vi "Quick Start - Runs - Get.vi"() -> ()   [LabVIEW 2020]
uses:
  Nominal Client/Nominal Client.lvclass
  19192e5f-c46e-4483-8f4d-33940d6cf31d.vi
  Run/Run.lvclass
panel:
  in  "runRid":string
  out "description":string
  out "Exists?":bool
  out "error out":errorcluster
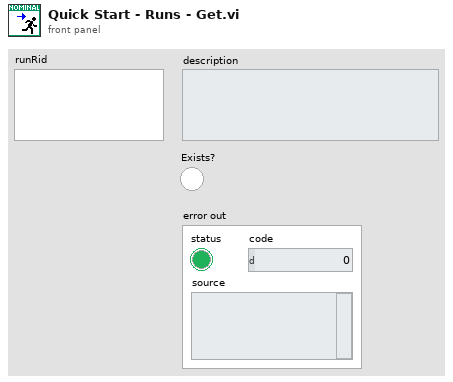
[diagram p1: front panel]
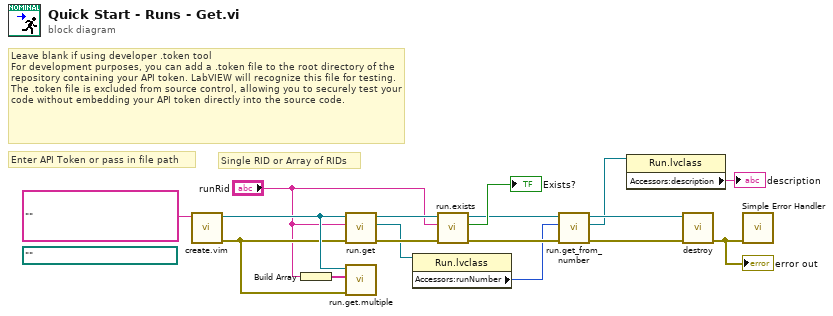
[diagram p0: block diagram]
diagram:
  (unwired) path ""
  # "Single RID or Array of RIDs"
  # "Leave blank if using developer .token tool\nFor development purposes, you can add a .token file to the root directory of the repository containing your API token. LabVIEW will recognize this file for testing. The .token file is excluded from source control, allowing you to securely test your code without embedding your API token directly into the source code."
  # "Enter API Token or pass in file path"
  n1 = call "create.vim"("API Token (string or path)"="" ("API Token")) -> ("error out"=w6:errorcluster, "Nominal Client"=w7:refnum<class "Nominal Client.lvclass">)  [unwired: 9 in]
  n2 = Build Array("runRid") -> (w2:string[])
  n3 = call "run.get.vi"("error in"=w6, "Run RID"="runRid", "Nominal Client in"=w7) -> ("error out"=w5:errorcluster, "Run"=w4:refnum<class "Run.lvclass">, "Nominal Client out"=w3:refnum<class "Nominal Client.lvclass">)  [unwired: 6 in]
  n4 = call "run.get.multiple.vi"("error in"=w6, "rid(s)"=w2, "Nominal Client in"=w7) -> ()  [unwired: 6 in, 3 out]
  n5 = property class="Run.lvclass"(reference=w4) -> ("Accessors:runNumber"=w10:i32)  [unwired: 1 in, 2 out]
  n6 = call "run.exists.vi"("error in"=w5, "RunRid"="runRid", "Nominal Client in"=w3) -> ("error out"=w13:errorcluster, "Exists?"=→"Exists?":bool, "Nominal Client out"=w14:refnum<class "Nominal Client.lvclass">)  [unwired: 6 in]
  n7 = call "run.get_from_number.vi"("error in"=w13, "Run Number"=w10, "Nominal Client in"=w14) -> ("error out"=w12:errorcluster, "Run"=w9:refnum<class "Run.lvclass">, "Nominal Client out"=w11:refnum<class "Nominal Client.lvclass">)  [unwired: 6 in]
  n8 = property class="Run.lvclass"(reference=w9) -> ("Accessors:description"=→"description":string)  [unwired: 1 in, 2 out]
  n9 = call "destroy.vi"("error in"=w12, "Nominal Client"=w11) -> ("error out"=w16:errorcluster)  [unwired: 9 in]
  "error out" <- w16
  n10 = call <vilib>:"Simple Error Handler.vi"("error in (no error)"=w16) -> ()  [unwired: 4 in, 5 out]
